vi "FEA_Model_Node-Meter_Converter.vi"(7 "Conversion Mode":T1(ring)=enum."Scalar Node to Meter", 8 "error in (no error)":errorcluster, 9 "Scalar in":dbl=0.06625781893205798, 10 "Array in":dbl[](array[numeric]), 11 "FEA_Model in":refnum<class "FEA_Model.lvclass">=refnum) -> (0 "error out":errorcluster, 1 "Scalar out":dbl, 2 "Array out":dbl[](array[numeric]), 3 "FEA_Model out":refnum<class "FEA_Model.lvclass">)   [LabVIEW 2021, in "FEA_Model.lvclass"]
uses:
  FEA_Model.lvclass
  FEA_Model.lvclass/FEA_Model.ctl
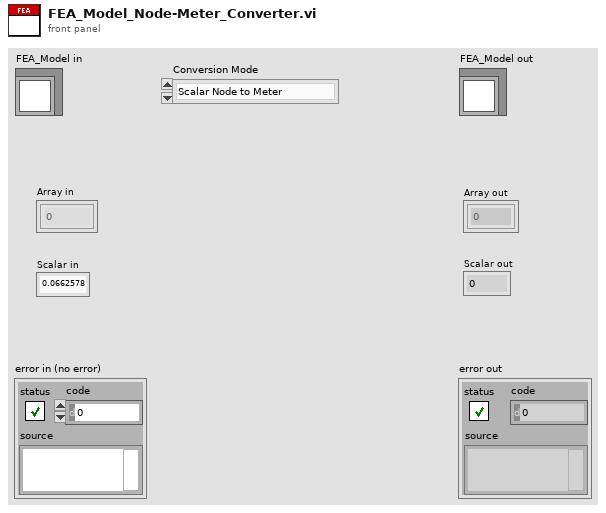
[diagram p1: front panel]
types:
  T1 = enum16{"Scalar Particle to Meter", "Scalar Node to Meter", "Scalar Meter to Particle", "Scalar Meter to Node", "Array Particle to Meter", "Array Node to Meter", "Array Meter to Particle", "Array Meter to Node"}
  T2 = enum16{"Particles to Nodes", "Particle to Node", "Nodes to Particles", "Node to Particle"}
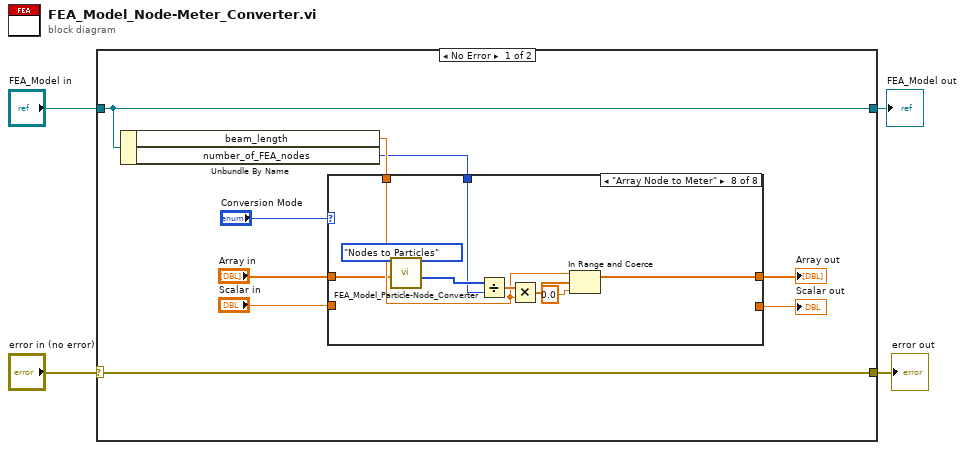
[diagram p0: block diagram]
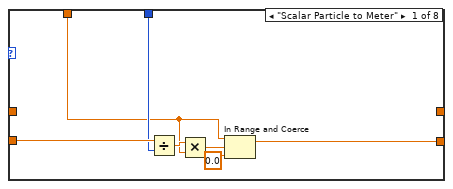
[diagram p2: hidden frame]
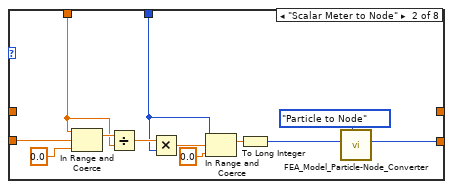
[diagram p3: hidden frame]
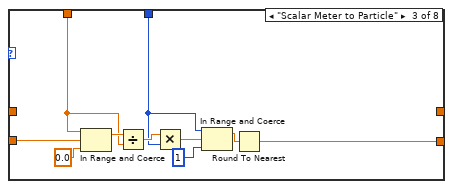
[diagram p4: hidden frame]
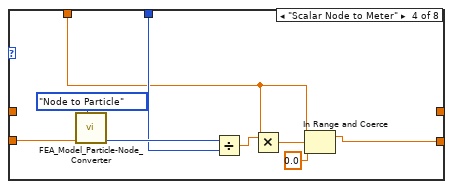
[diagram p5: hidden frame]
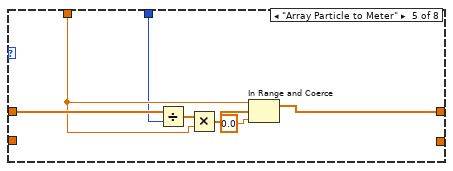
[diagram p6: hidden frame]
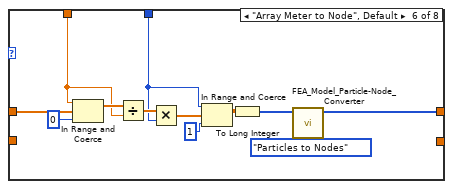
[diagram p7: hidden frame]
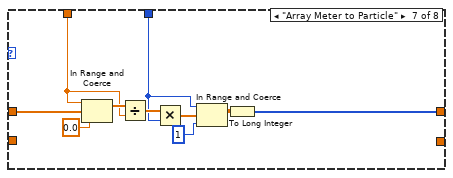
[diagram p8: hidden frame]
diagram:
  n1 = case shown="No Error" "error in (no error)" {
    selector: "error in (no error)" -> [w13 w91]
    tunnel: [w13 w91] -> w3
    tunnel: [w12 w90] -> w1
    tunnel: "FEA_Model in" -> [w12 w90]
    frame No Error {
      n2 = Unbundle By Name(w12) -> ("beam_length"=w6:dbl, "number_of_FEA_nodes"=w5:i32)
      n3 = case shown="\"Array Node to Meter\"" "Conversion Mode" {
        tunnel: "Array in" -> [_ _ _ _ w55 w64 w74 w81]
        tunnel: "Scalar in" -> [w17 w26 w36 w47 _ _ _ _]
        tunnel: [_ _ _ _ w54 w61 w73 w89] -> w8
        tunnel: [w16 w23 w35 w48 _ _ _ _] -> w9
        tunnel: w6 -> [w14 w22 w34 w43 w53 w60 w72 w82]
        tunnel: w5 -> [w15 w21 w33 w44 w52 w59 w71 w83]
        frame "Scalar Particle to Meter" {
          n4 = Divide(x=w17, y=w15) -> (x/y=w19:dbl)
          n5 = Multiply(x=w19, y=w14) -> (x*y=w18:dbl)
          n6 = In Range and Coerce(upper limit=w14, x=w18, lower limit=0.0) -> (coerced(x)=w16:dbl)  [unwired: 1 out]
        }
        frame "Scalar Meter to Node" {
          n7 = In Range and Coerce(upper limit=w22, x=w26, lower limit=0.0) -> (coerced(x)=w28:dbl)  [unwired: 1 out]
          n8 = Divide(x=w28, y=w22) -> (x/y=w31:dbl)
          n9 = Multiply(x=w31, y=w21) -> (x*y=w30:dbl)
          n10 = In Range and Coerce(upper limit=w21, x=w30, lower limit=0.0) -> (coerced(x)=w32:dbl)  [unwired: 1 out]
          n11 = To Long Integer(number=w32) -> (32bit integer=w24:i32)
          n12 = call "FEA_Model_Particle-Node_Converter.vi"("mode"=T2."Particle to Node", "Particle"=w24) -> ("Node"=w23:i32)  [unwired: 6 in, 3 out]
        }
        frame "Scalar Meter to Particle" {
          n13 = In Range and Coerce(upper limit=w34, x=w36, lower limit=0.0) -> (coerced(x)=w38:dbl)  [unwired: 1 out]
          n14 = Divide(x=w38, y=w34) -> (x/y=w41:dbl)
          n15 = Multiply(x=w41, y=w33) -> (x*y=w40:dbl)
          n16 = In Range and Coerce(upper limit=w33, x=w40, lower limit=1) -> (coerced(x)=w42:dbl)  [unwired: 1 out]
          n17 = Round To Nearest(number=w42) -> (nearest integer value=w35:dbl)
        }
        frame "Scalar Node to Meter" {
          n18 = call "FEA_Model_Particle-Node_Converter.vi"("mode"=T2."Node to Particle", "Node"=w47) -> ("Particle"=w45:i32)  [unwired: 6 in, 3 out]
          n19 = Divide(x=w45, y=w44) -> (x/y=w50:dbl)
          n20 = Multiply(x=w50, y=w43) -> (x*y=w49:dbl)
          n21 = In Range and Coerce(upper limit=w43, x=w49, lower limit=0.0) -> (coerced(x)=w48:dbl)  [unwired: 1 out]
        }
        frame "Array Particle to Meter" {
          n22 = Divide(x=w55, y=w52) -> (x/y=w57:dbl[])
          n23 = Multiply(x=w57, y=w53) -> (x*y=w56:dbl[])
          n24 = In Range and Coerce(upper limit=w53, x=w56, lower limit=0.0) -> (coerced(x)=w54:dbl[])  [unwired: 1 out]
        }
        frame "Array Meter to Node", Default {
          n25 = In Range and Coerce(upper limit=w60, x=w64, lower limit=0) -> (coerced(x)=w66:dbl[])  [unwired: 1 out]
          n26 = Divide(x=w66, y=w60) -> (x/y=w69:dbl[])
          n27 = Multiply(x=w69, y=w59) -> (x*y=w68:dbl[])
          n28 = In Range and Coerce(upper limit=w59, x=w68, lower limit=1) -> (coerced(x)=w70:dbl[])  [unwired: 1 out]
          n29 = To Long Integer(number=w70) -> (32bit integer=w63:i32[])
          n30 = call "FEA_Model_Particle-Node_Converter.vi"("mode"=T2."Particles to Nodes", "Particles"=w63) -> ("Nodes"=w61:i32[])  [unwired: 6 in, 3 out]
        }
        frame "Array Meter to Particle" {
          n31 = In Range and Coerce(upper limit=w72, x=w74, lower limit=0.0) -> (coerced(x)=w76:dbl[])  [unwired: 1 out]
          n32 = Divide(x=w76, y=w72) -> (x/y=w79:dbl[])
          n33 = Multiply(x=w79, y=w71) -> (x*y=w78:dbl[])
          n34 = In Range and Coerce(upper limit=w71, x=w78, lower limit=1) -> (coerced(x)=w80:dbl[])  [unwired: 1 out]
          n35 = To Long Integer(number=w80) -> (32bit integer=w73:i32[])
        }
        frame "Array Node to Meter" {
          n36 = call "FEA_Model_Particle-Node_Converter.vi"("mode"=T2."Nodes to Particles", "Nodes"=w81) -> ("Particles"=w84:i32[])  [unwired: 6 in, 3 out]
          n37 = Divide(x=w84, y=w83) -> (x/y=w87:dbl[])
          n38 = Multiply(x=w87, y=w82) -> (x*y=w86:dbl[])
          n39 = In Range and Coerce(upper limit=w82, x=w86, lower limit=0.0) -> (coerced(x)=w89:dbl[])  [unwired: 1 out]
        }
      }
      "Array out" <- w8
      "Scalar out" <- w9
    }
    frame Error {
    }
  }
  "error out" <- w3
  "FEA_Model out" <- w1
